vi "Write Volume.vi"(8 "error in (no error)":errorcluster, 10 "Volume":dbl, 11 "Channel in":refnum<data-value>) -> (0 "error out":errorcluster, 3 "Channel out":refnum<data-value>)   [LabVIEW 2020, in "G-Audio.lvlib" / "Channel.lvclass"]
uses:
  Channel.lvclass
  Channel.lvclass/Channel.ctl
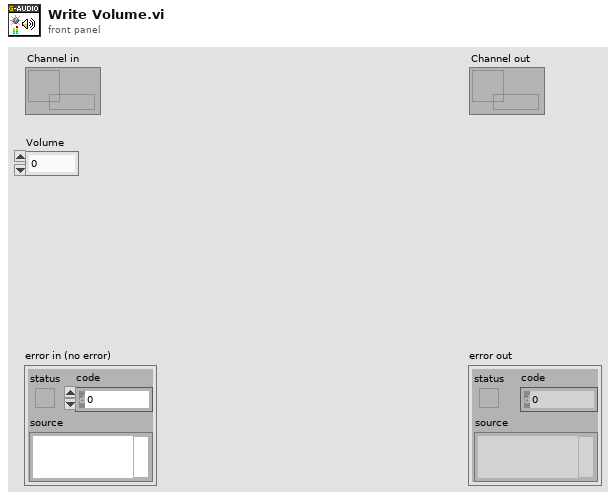
[diagram p1: front panel]
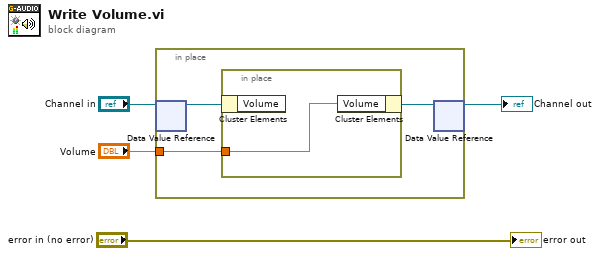
[diagram p0: block diagram]
diagram:
  n1 = in-place {
    in-place-border: "Volume" -> [w5]
    n2 = in-place-dvr #1("Channel in") -> (w7:refnum<class "Channel.lvclass">)  [unwired: 1 out]
    n3 = in-place {
      in-place-border: w5 -> [w8]
      n4 = in-place-cluster #2(w7) -> ()  [unwired: 1 out]
      n5 = in-place-cluster #2("Volume"=w8) -> (w6:refnum<class "Channel.lvclass">)
    }
    n6 = in-place-dvr #1(w6) -> (→"Channel out":refnum<data-value>)  [unwired: 1 out]
  }
  "error out" <- "error in (no error)"
